vi "Mod_OFDM_Block_IFFT_per_Frame.vi"(0 "Complex Mapping":cdb[][](array[numeric]), 7 "Parameters per Ofdm Symbol":T1 {"Data Source"."Data Source"."Register Initial State" format="%08x"}, 11 "error in (no error)":errorcluster) -> (4 "IFFT Out":cdb[][](array[numeric]), 8 "Parameters per Ofdm Symbol":T1 {"Data Source"."Data Source"."Register Initial State" format="%08x"}, 15 "error out":errorcluster)   [LabVIEW 2010]
doc: "Block IFFT is performed on the complex signal\n\nNote: The common way to implement the inverse Fourier transform is by an inverse Fast Fourier Transform (IFFT). If, for example, a 64-point IFFT is used, the coefficients 0 to +31 are mapped to the same numbered IFFT inputs, while the coefficients -32 to -1 are copied into IFFT inputs +32 to +63."
uses:
  Controls(Type_DEf)/Parameters per Ofdm Symbol.ctl
  <vilib>/Analysis/2dsp.llb/Inverse Complex FFT.vi
  <vilib>/Analysis/NI_AALPro.lvlib
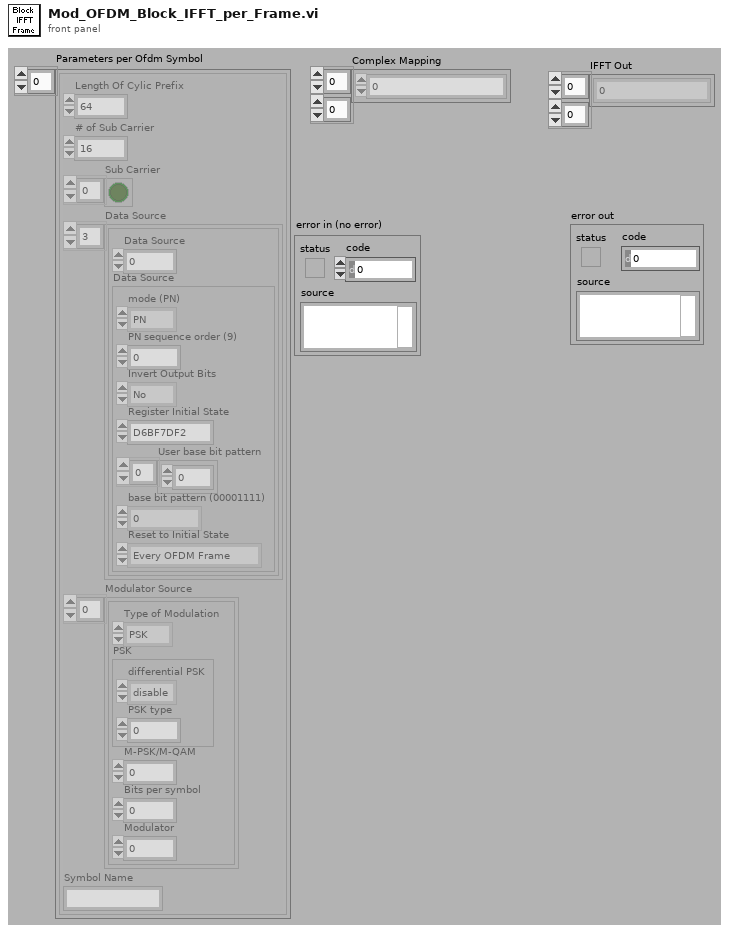
[diagram p1: front panel]
types:
  T1 = typedef "Parameters per Ofdm Symbol.ctl" = cluster{"Length Of Cylic Prefix":i32, "# of Sub Carrier":i32, "Sub Carrier":bool[], "Data Source":cluster{"Data Source":u16, "Data Source":cluster{"mode (PN)":enum16{"PN", "pattern", "user"}, "PN sequence order (9)":i32, "Invert Output Bits":enum16{"No", "Yes"}, "Register Initial State":u32, "User base bit pattern":i8[], "base bit pattern (00001111)":enum16{"0", "1", "01", "0011", "00001111"}, "Reset to Initial State":enum16{"Every OFDM Frame", "Every OFDM Symbol", "Every Sub Carrier"}}}[], "Modulator Source":cluster{"Type of Modulation":enum16{"PSK", "QAM"}, "PSK":cluster{"differential PSK":enum16{"disable", "enable"}, "PSK type":u16}, "M-PSK/M-QAM":i32, "Bits per symbol":i32, "Modulator":u16}[], "Symbol Name":string}[]
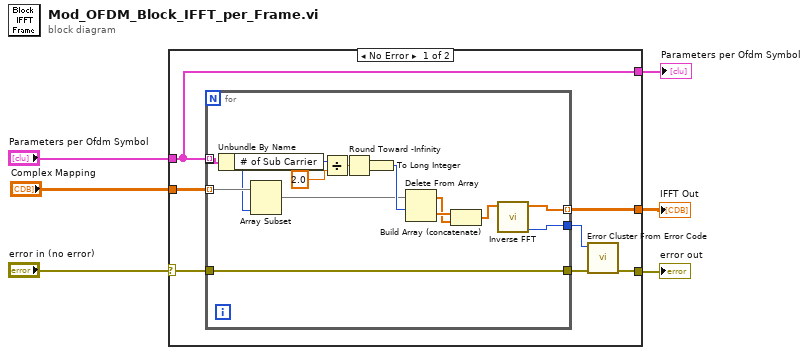
[diagram p0: block diagram]
diagram:
  n1 = case shown="No Error" "error in (no error)" {
    selector: "error in (no error)" -> [w8 w28]
    tunnel: "Complex Mapping" -> [w13 _]
    tunnel: [w12 _] -> w5
    tunnel: "Parameters per Ofdm Symbol" -> [w11 _]
    tunnel: [w11 _] -> w2
    tunnel: [w9 w28] -> w1
    frame No Error {
      n2 = for {
        tunnel: w13 -> [w25] mode=indexing
        tunnel: [w27] -> w12 mode=indexing
        tunnel: [w26] -> _ mode=indexing
        tunnel: w11 -> [w26] mode=indexing
        tunnel: [w24] -> w10
        tunnel: w8 -> [w16]
        tunnel: [w16] -> w7
        n3 = Unbundle By Name(w26) -> ("# of Sub Carrier"=w21:i32)
        n4 = Array Subset(array=w25, length=w21) -> (w15:cdb[])  [unwired: 1 in]
        n5 = Divide(x=w21, y=2.0) -> (x/y=w19:dbl)
        n6 = Round Toward -Infinity(1:w19) -> (0:w18:dbl)
        n7 = To Long Integer(number=w18) -> (32bit integer=w17:i32)
        n8 = Delete From Array(array=w15, length=w17) -> (deleted portion=w23:cdb[], array with subset deleted=w22:cdb[])  [unwired: 1 in]
        n9 = Build Array (concatenate)(w23, w22) -> (w14:cdb[])
        n10 = call-poly <vilib>:"Inverse FFT.vi"("FFT {X}"=w14) -> ("error"=w24:i32, "X"=w27:cdb[])  [unwired: 9 in]
      }
      n11 = call <vilib>:"Error Cluster From Error Code.vi"("error in (no error)"=w7, "error code (0)"=w10) -> ("error out"=w9:errorcluster)  [unwired: 7 in]
    }
    frame Error {
    }
  }
  "IFFT Out" <- w5
  "error out" <- w1
  "Parameters per Ofdm Symbol" <- w2
